vi "rs3 free error.vi"(8 "error in (no error)":errorcluster, 11 "error in":u64) -> (0 "error out 2":errorcluster, 3 "error out":u64)   [LabVIEW 2018, in "libRealSense3.lvlib"]
doc: "void rs_free_error (rs_error * error);"
uses:
  libRealSense3.lvlib
  realsense2.dll
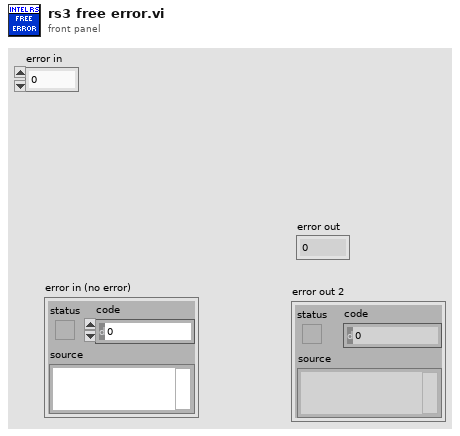
[diagram p1: front panel]
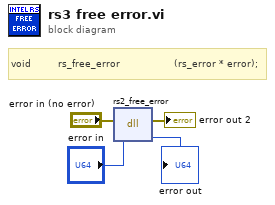
[diagram p0: block diagram]
diagram:
  # "void         rs_free_error                  (rs_error * error);"
  n1 = dll-call lib="C:/Users/aaron.jencks/Documents/Temp/realsense_labview_sdk/RealSense SDK2.11.0 for LabVIEW/realsense2.dll" fn="rs2_free_error"(error in="error in (no error)", "error"="error in") -> (error out=→"error out 2":errorcluster, "error"=→"error out":u64)  [unwired: 3 in, 1 out]
